vi "CO-ORD.vi"(2 "Y":i32, 3 "X":i32, 4 "ANGLE":T1=2 items=["0", "45", "90", "135", "180", "225", "270", "315"], 5 "Add?":bool) -> (0 "Y OUT":i32, 1 "X OUT":i32)   [LabVIEW 2014]
uses:
  Controls/Direction enum.ctl
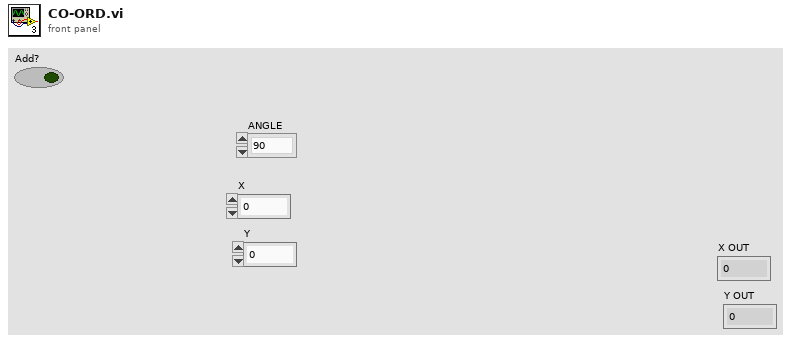
[diagram p1: front panel]
types:
  T1 = typedef "Direction enum.ctl" = u16
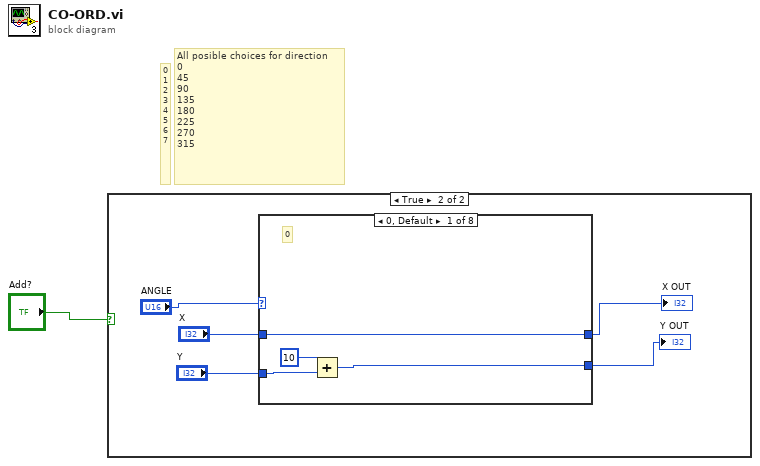
[diagram p0: block diagram]
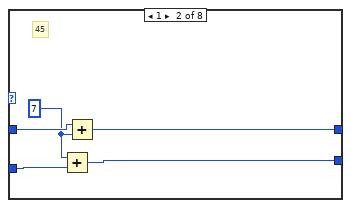
[diagram p3: hidden frame]
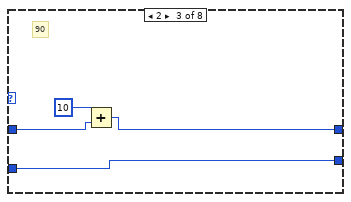
[diagram p4: hidden frame]
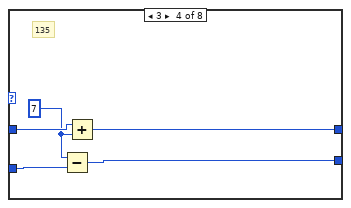
[diagram p5: hidden frame]
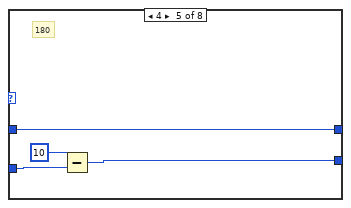
[diagram p6: hidden frame]
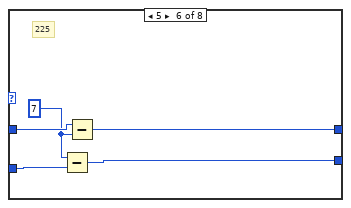
[diagram p7: hidden frame]
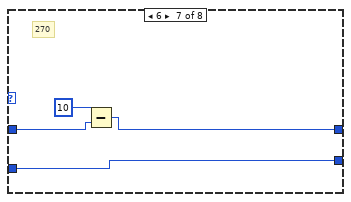
[diagram p8: hidden frame]
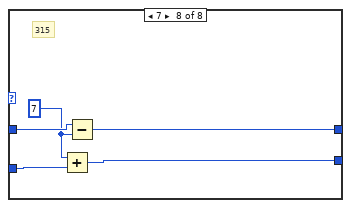
[diagram p9: hidden frame]
diagram:
  # "0\n1\n2\n3\n4\n5\n6\n7"
  # "All posible choices for direction\n0\n45\n90\n135\n180\n225\n270\n315"
  n1 = case shown="True" "Add?" {
    frame False {
    }
    frame True {
      n2 = case shown="0, Default" "ANGLE" {
        tunnel: "X" -> [w7 w13 w18 w22 w25 w31 w36 w40]
        tunnel: "Y" -> [w10 w15 w16 w24 w28 w33 w34 w42]
        tunnel: [w8 w14 w16 w23 w26 w32 w34 w41] -> w3
        tunnel: [w7 w11 w17 w20 w25 w29 w35 w38] -> w2
        frame 0, Default {
          # "0"
          n3 = Add(x=10, y=w10) -> (x+y=w8:i32)
        }
        frame 1 {
          w12 = 7
          # "45"
          n4 = Add(x=w12, y=w15) -> (x+y=w14:i32)
          n5 = Add(x=w13, y=w12) -> (x+y=w11:i32)
        }
        frame 2 {
          # "90"
          n6 = Add(x=10, y=w18) -> (x+y=w17:i32)
        }
        frame 3 {
          w21 = 7
          # "135"
          n7 = Subtract(x=w21, y=w24) -> (x-y=w23:i32)
          n8 = Add(x=w22, y=w21) -> (x+y=w20:i32)
        }
        frame 4 {
          # "180"
          n9 = Subtract(x=10, y=w28) -> (x-y=w26:i32)
        }
        frame 5 {
          w30 = 7
          # "225"
          n10 = Subtract(x=w30, y=w33) -> (x-y=w32:i32)
          n11 = Subtract(x=w31, y=w30) -> (x-y=w29:i32)
        }
        frame 6 {
          # "270"
          n12 = Subtract(x=10, y=w36) -> (x-y=w35:i32)
        }
        frame 7 {
          w39 = 7
          # "315"
          n13 = Add(x=w39, y=w42) -> (x+y=w41:i32)
          n14 = Subtract(x=w40, y=w39) -> (x-y=w38:i32)
        }
      }
      "X OUT" <- w2
      "Y OUT" <- w3
    }
  }
